vi "Process Job.vi"(8 "error in (no error)":errorcluster, 10 "Job":refnum<class>, 11 "Process Job In":refnum<class "Job Handler.lvclass">) -> (0 "error out":errorcluster, 3 "Process Job Out":refnum<class "Job Handler.lvclass">)   [LabVIEW 2020, in "Job Handler.lvclass"]
uses:
  Job Handler.lvclass
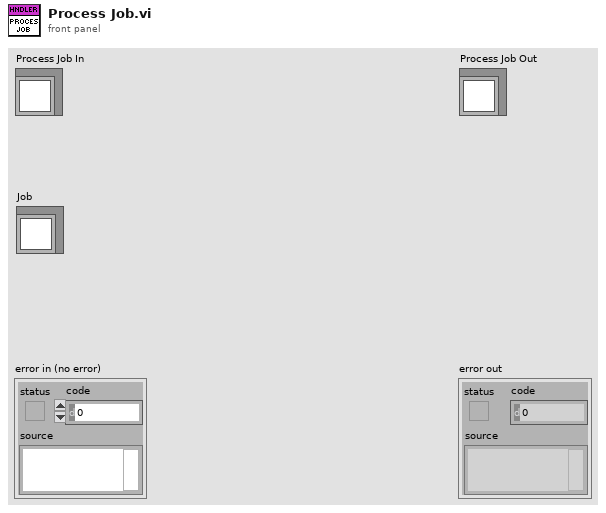
[diagram p1: front panel]
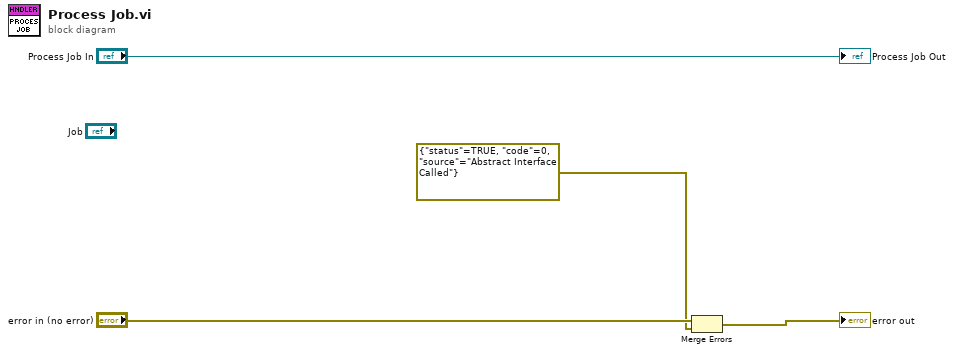
[diagram p0: block diagram]
diagram:
  n1 = Merge Errors("error in (no error)", errorcluster {"status"=TRUE, "code"=0, "source"="Abstract Interface Called"} ("error in (no error)")) -> (→"error out":errorcluster)
  "Process Job Out" <- "Process Job In"
